vi "Activate CPY.vi"(5 "DO Task":refnum<k21>, 7 "AO Task":refnum<k21>, 8 "error in (no error)":errorcluster, 10 "AO":T1(array[cluster]), 11 "DO":T2(array[cluster])=[{"CDT"=-150.0, "Position"=TRUE, "Component ID"="F_EPV_131"}, {"CDT"=-150.0, "Position"=TRUE, "Component ID"="F_EPV_131"}, {"CDT"=-135.0, "Position"=FALSE, "Component ID"="F_EPV_132"}, {"CDT"=-120.0, "Position"=FALSE, "Component ID"="F_EPV_131"}, {"CDT"=-20.0, "Position"=TRUE, "Component ID"="F_EPV_136"}, {"CDT"=-10.0, "Position"=FALSE, "Component ID"="F_EPV_136"}]) -> (0 "error out":errorcluster, 3 "Abort":bool)   [LabVIEW 2022 SP3]
uses:
  <vilib>/platform/TimedLoop/XDataNode/XDataNode.xnode
  <vilib>/Platform/TimedLoop/XDataNode/nitl_modes.ctl
  <vilib>/Platform/TimedLoop/XDataNode/XDNodeRunTimeDep.lvlib
  <vilib>/Platform/TimedLoop/XDataNode/wakeup.ctl
  <vilib>/Platform/TimedLoop/XDataNode/timing_clust.ctl
  RT Sub VI's/RT Global.vi
  <vilib>/DAQmx/write.llb/DAQmx Write (Digital 1D Bool NChan 1Samp 1Line).vi
  <vilib>/DAQmx/write.llb/DAQmx Write (Analog 1D DBL 1Chan NSamp).vi
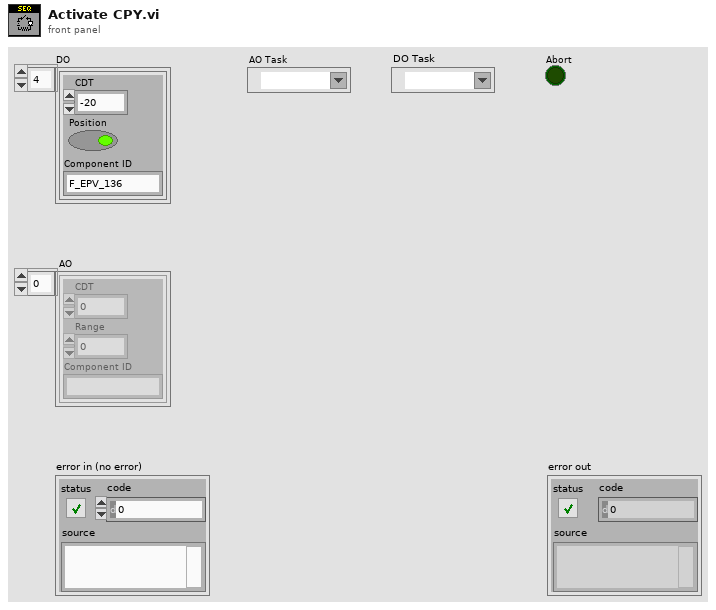
[diagram p1: front panel]
types:
  T1 = cluster{"CDT":dbl, "Range":dbl, "Component ID":string}[]
  T2 = cluster{"CDT":dbl, "Position":bool, "Component ID":string}[]
  T3 = typedef "RT All Queue.ctl" = cluster{"AI\nAO\nDO\nTC\nACC\nStrain":refnum<queue>[], "DI":refnum<queue>}
  T4 = cluster{"AO":cluster{"CDT":dbl, "Range":dbl, "Component ID":string}[], "DO":cluster{"CDT":dbl, "Position":bool, "Component ID":string}[], "Launch Time":timestamp}
  T5 = typedef "XDNodeRunTimeDep.lvlib/timing_clust.ctl" = cluster{"Expected End [f-1]":u64, "Actual End [f-1]":u64, "Finished Late? [f-1]":bool, "Expected End [i-1]":u64, "Actual End [i-1]":u64, "Finished Late? [i-1]":bool, "Expected Start [i]":u64, "Actual Start [i]":u64, "Expected Start [f]":u64, "Actual Start [f]":u64, "Source Name":string, "Structure Name":string, "Period":i64, "Deadline":i64, "Offset":i64, "Start":i64, "Priority":i32, "Timeout":i32, "Mode":T6, "Wakeup Reason":T7, "Error":errorcluster, "Source Type":string, "Secondary Source Type":string, "Global End Time":u64, "Global Start Time":u64, "Frame Duration":u64, "Iteration Duration":u64, "Assigned CPU":i32, "I/O Scan Engine Mode":u32}
  T6 = typedef "XDNodeRunTimeDep.lvlib/nitl_modes.ctl" = enum32{"No Change", "Process missed periods, maintain original phase", "Discard missed periods, maintain original phase", "Process missed periods, ignore original phase", "Discard missed periods, ignore original phase"}
  T7 = typedef "XDNodeRunTimeDep.lvlib/wakeup.ctl" = enum32{"Normal", "Aborted", "Asynchronous wakeup", "Timing source error", "Timed loop error", "Timeout"}
  T8 = cluster{"CDT":dbl, "Position":bool, "Component ID":string}
  T9 = cluster{"CDT":dbl, "Range":dbl, "Component ID":string}
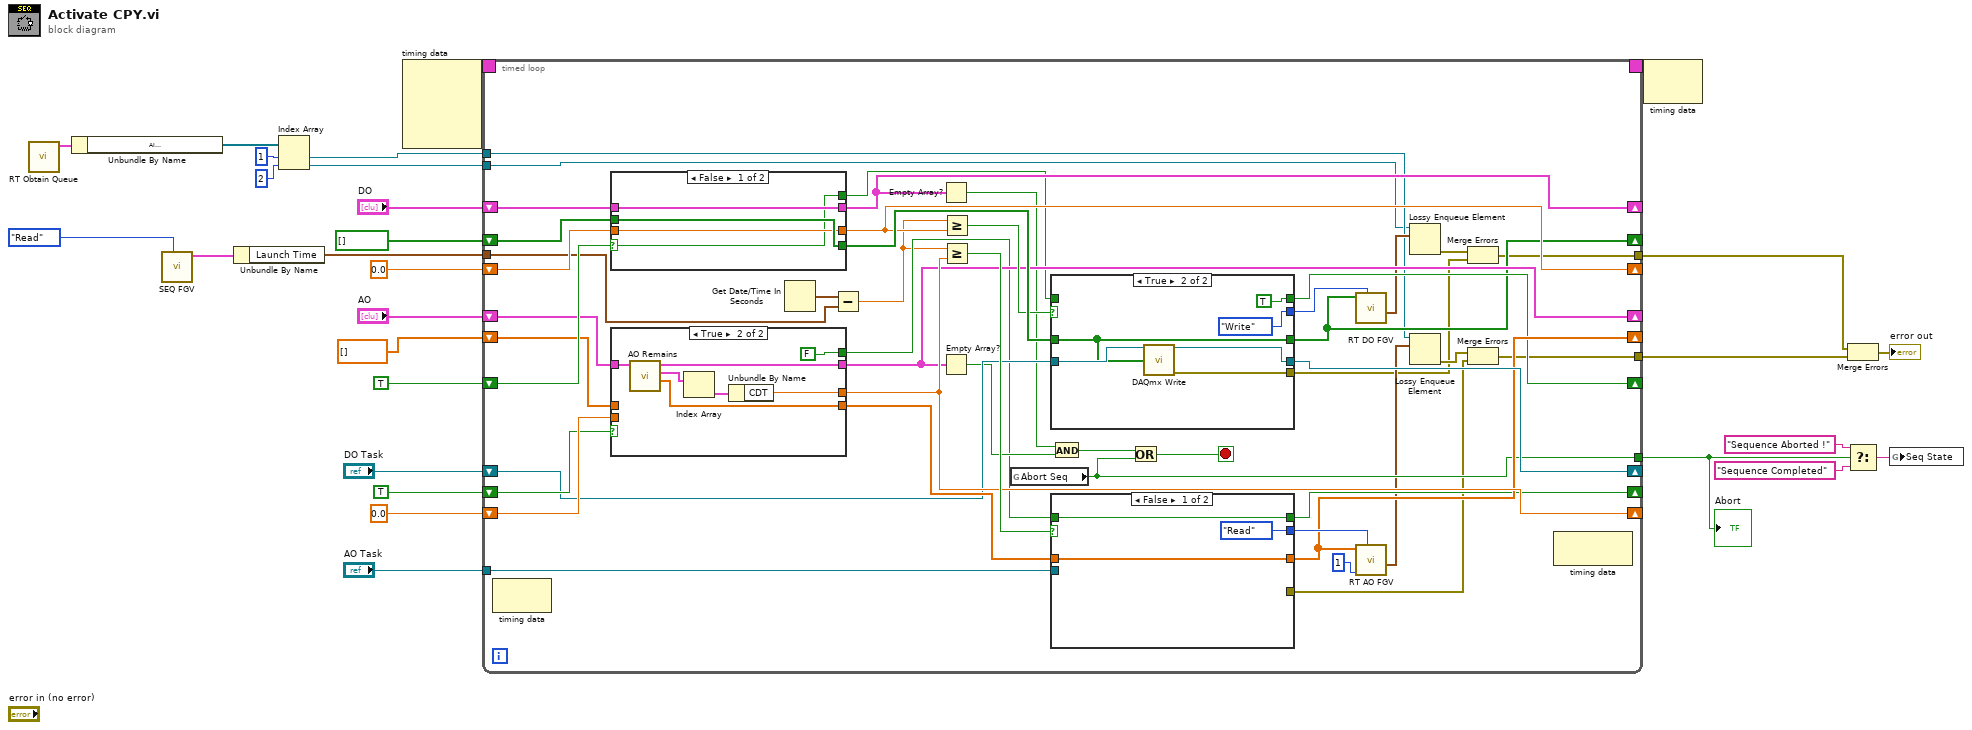
[diagram p0: block diagram]
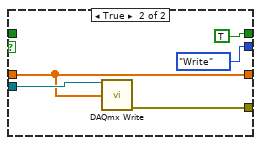
[diagram p2: hidden frame]
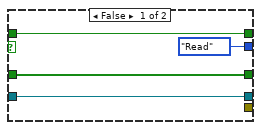
[diagram p4: hidden frame]
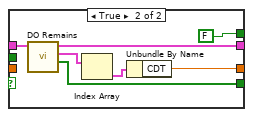
[diagram p5: hidden frame]
diagram:
  n1 = call "RT Obtain Queue.vi"() -> ("Queue ref"=w7:T3)  [unwired: 10 in, 1 out]
  n2 = Unbundle By Name(w7) -> ("AI\nAO\nDO\nTC\nACC\nStrain"=w6:refnum<queue>[])
  n3 = call "SEQ FGV.vi"("Enum"=enum16{"Read", "Write"}."Read") -> ("Seq data out"=w18:T4)  [unwired: 9 in, 1 out]
  n4 = Unbundle By Name(w18) -> ("Launch Time"=w17:timestamp)
  n5 = Index Array(array=w6, index #1=1 ("index"), index #2=2 ("index")) -> (element #1=w3:refnum<queue>, element #2=w2:refnum<queue>)
  n6 = node-c288() -> (w21:T5)  [unwired: 4 in]
  n7 = timed-loop {
    shift-right: [w50] -> _
    shift-left: "DO" -> [w74]
    shift-right: [w45] -> _
    shift-left: TRUE -> [w73]
    shift-right: [w41] -> _
    shift-left: bool[] [] ("DO value") -> [w72]
    shift-right: [w68] -> _
    shift-left: 0.0 ("CDT") -> [w71]
    shift-right: [w64] -> _
    shift-left: 0.0 ("CDT") -> [w67]
    shift-right: [w53] -> _
    shift-left: "AO" -> [w66]
    shift-right: [w43] -> _
    shift-left: TRUE -> [w62]
    shift-right: [w55] -> _
    shift-left: dbl[] [] ("AO") -> [w61]
    shift-right: [w59] -> _
    shift-left: "DO Task" -> [w60]
    tunnel: [w34] -> w24
    tunnel: "AO Task" -> [w58]
    tunnel: [w39] -> w9
    timing: w21 -> [_]
    timing-out: [_] -> w20
    tunnel: w17 -> [w51]
    tunnel: [w31] -> w8
    tunnel: w3 -> [w30]
    tunnel: w2 -> [w29]
    stop <- w54 stop-if-true
    n8 = node-c288() -> ()  [unwired: 1 in, 1 out]
    n9 = case shown="False" w73 {
      selector: w73 -> [w106 _]
      tunnel: w74 -> [w107 w116]
      tunnel: [w107 w111] -> w50
      tunnel: [w109 w113] -> w70
      tunnel: w72 -> [w109 _]
      tunnel: [w108 w112] -> w68
      tunnel: w71 -> [w108 _]
      tunnel: [w106 FALSE] -> w46
      frame False {
      }
      frame True {
        n10 = call "DO Remains.vi"("Array"=w116) -> ("DO value"=w113:bool[], "Same DO"=w115:T2, "Remains"=w111:T2)  [unwired: 7 in, 1 out]
        n11 = Index Array(array=w115) -> (element=w114:T8)  [unwired: 1 in]
        n12 = Unbundle By Name(w114) -> ("CDT"=w112:dbl)
      }
    }
    n13 = case shown="True" w62 {
      selector: w62 -> [w86 _]
      tunnel: w66 -> [w87 w95]
      tunnel: [w87 w91] -> w53
      tunnel: [w88 w92] -> w64
      tunnel: w67 -> [w88 _]
      tunnel: [w86 FALSE] -> w44
      tunnel: [w85 w89] -> w63
      tunnel: w61 -> [w85 _]
      frame False {
      }
      frame True {
        n14 = call "AO Remains.vi"("Array"=w95) -> ("AO"=w89:dbl[], "Same AO"=w94:T1, "Remains AO"=w91:T1)  [unwired: 7 in, 1 out]
        n15 = Index Array(array=w94) -> (element=w93:T9)  [unwired: 1 in]
        n16 = Unbundle By Name(w93) -> ("CDT"=w92:dbl)
      }
    }
    n17 = Get Date/Time In Seconds() -> (seconds since 1Jan1904=w52:timestamp)
    n18 = Subtract(x=w52, y=w51) -> (x-y=w42:dbl)
    n19 = Empty Array?(array=w50) -> (empty?=w49:bool)
    n20 = Empty Array?(array=w53) -> (empty?=w48:bool)
    n21 = Greater Or Equal?(x=w42, y=w68) -> (x >= y?=w69:bool)
    n22 = Greater Or Equal?(x=w42, y=w64) -> (x >= y?=w65:bool)
    n23 = global read "RT Global.vi" "Abort Seq"() -> (w39:bool)
    n24 = case shown="True" w69 {
      tunnel: w70 -> [w99 w103]
      tunnel: [w99 w103] -> w41
      tunnel: w60 -> [w98 w105]
      tunnel: [w98 w104] -> w59
      tunnel: [_ w102] -> w32
      tunnel: [enum16{"Read", "Write", "Start time", "init"}."Read" ("Enum") enum16{"Read", "Write", "Start time", "init"}."Write" ("Enum")] -> w57
      tunnel: w46 -> [w96 _]
      tunnel: [w96 TRUE] -> w45
      frame False {
      }
      frame True {
        n25 = call-poly <vilib>:"DAQmx Write.vi"("task/channels in"=w105, "data"=w103) -> ("task out"=w104:refnum<k21>, "error out"=w102:errorcluster)  [unwired: 11 in, 1 out]
      }
    }
    n26 = case shown="False" w65 {
      tunnel: w63 -> [w78 w81]
      tunnel: [w78 w81] -> w55
      tunnel: [_ w84] -> w35
      tunnel: w58 -> [_ w83]
      tunnel: [enum16{"Read", "Write", "Start time", "init"}."Read" ("Enum") enum16{"Read", "Write", "Start time", "init"}."Write" ("Enum")] -> w56
      tunnel: w44 -> [w77 _]
      tunnel: [w77 TRUE] -> w43
      frame False {
      }
      frame True {
        n27 = call-poly <vilib>:"DAQmx Write.vi"("task/channels in"=w83, "data"=w81) -> ("error out"=w84:errorcluster)  [unwired: 11 in, 2 out]
      }
    }
    n28 = And(x=w49, y=w48) -> (x .and. y?=w47:bool)
    n29 = Or(x=w47, y=w39) -> (x .or. y?=w54:bool)
    n30 = call "RT DO FGV.vi"("Enum"=w57, "DO in"=w41) -> ("DO Waveform"=w38:waveform(dbl)[])  [unwired: 7 in, 2 out]
    n31 = call "RT AO FGV.vi"("Enum"=w56, "Size"=1, "AO in"=w55) -> ("AO Waveform"=w37:waveform(dbl)[])  [unwired: 6 in, 2 out]
    n32 = Lossy Enqueue Element(queue=w29, element=w38) -> (error out=w33:errorcluster)  [unwired: 1 in, 3 out]
    n33 = Lossy Enqueue Element(queue=w30, element=w37) -> (error out=w36:errorcluster)  [unwired: 1 in, 3 out]
    n34 = Merge Errors(w33, w32) -> (w31:errorcluster)
    n35 = Merge Errors(w36, w35) -> (w34:errorcluster)
    n36 = node-c288() -> ()  [unwired: 1 in, 1 out]
  }
  "Abort" <- w9
  n37 = node-c288(w20) -> ()  [unwired: 1 out]
  n38 = Merge Errors(w8, w24) -> (→"error out":errorcluster)
  n39 = Select(t="Sequence Aborted !" ("Seq State"), s=w9, f="Sequence Completed" ("Seq State")) -> (s? t:f=w10:string)
  n40 = global write "RT Global.vi" "Seq State"(w10) -> ()
